vi "Get New Library Path.vi"(9 "Rename":string, 10 "Name Folder Path":path) -> (2 "New Library Path":path)   [LabVIEW 2021, in "_Rename.lvlib" / "_Rename.lvclass"]
uses:
  _Rename.lvclass
  _Rename.lvclass/_Rename.ctl
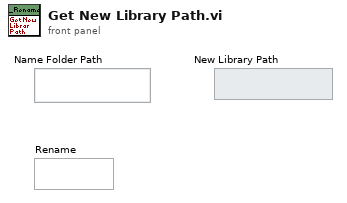
[diagram p1: front panel]
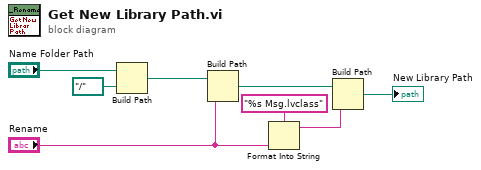
[diagram p0: block diagram]
diagram:
  n1 = Build Path(base path="Name Folder Path", name or relative path=path "../..") -> (appended path=w7:path)
  n2 = Build Path(base path=w7, name or relative path="Rename") -> (appended path=w6:path)
  n3 = Format Into String(format string="%s Msg.lvclass", "Rename") -> (resulting string=w4:string)  [unwired: 2 in, 1 out]
  n4 = Build Path(base path=w6, name or relative path=w4) -> (appended path=→"New Library Path":path)
